vi "Implode String.vi"(7 "Delimiter (Comma)":string=",", 11 "String Array":string[](array[string])) -> (3 "Delimited String":string)   [LabVIEW 2016, in "Better Search.lvlib"]
uses:
  Better Search.lvlib
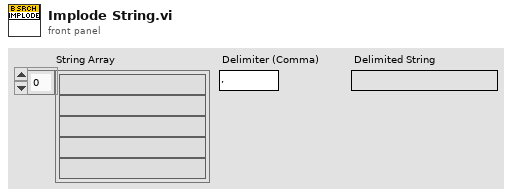
[diagram p1: front panel]
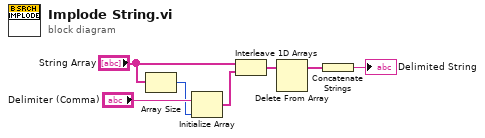
[diagram p0: block diagram]
diagram:
  n1 = Array Size(array="String Array") -> (size(s)=w6:i32)
  n2 = Initialize Array("Delimiter (Comma)", w6) -> (w4:string[])
  n3 = Interleave 1D Arrays("String Array", w4) -> (w3:string[])
  n4 = Delete From Array(array=w3) -> (array with subset deleted=w2:string[])  [unwired: 2 in, 1 out]
  n5 = Concatenate Strings(w2) -> (→"Delimited String":string)
